vi "Create Master Instance.vi"   [LabVIEW 2014, in "Modbus Master.lvclass"]
doc: "创建串口或TCPModbus主设备实例.必须手动选择所需多态实例。"
uses:
  <vilib>/Modbus/master/Modbus Master.lvclass
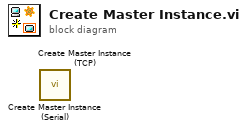
[diagram p0: block diagram]
diagram:
  n1 = call <vilib>:"Create Master Instance (Serial).vi"() -> ()  [unwired: 10 in, 2 out]
  n2 = call <vilib>:"Create Master Instance (TCP).vi"() -> ()  [unwired: 10 in, 2 out]
